vi "Write data file (SubVI).vi"(7 "format (%.;%.7e)":string="%.;%.7e", 8 "error in":errorcluster, 9 "Binary":bool, 10 "2D data":dbl[][](array[numeric]), 11 "file path in":path) -> (0 "error out":errorcluster, 3 "file path out":path)   [LabVIEW 2019]
doc: "Writes measurement data to a file (binary or text based)"
uses:
  <vilib>/Utility/file.llb/Write Delimited Spreadsheet (DBL).vi
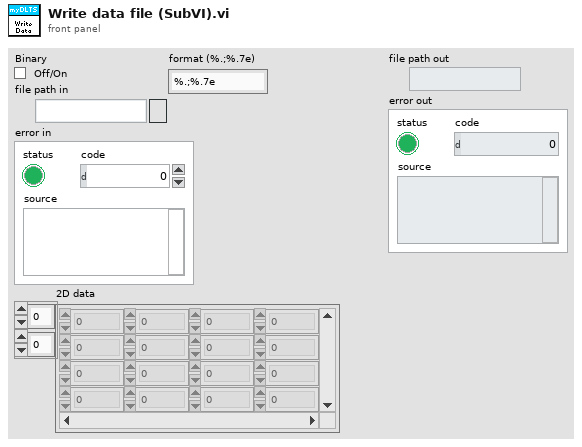
[diagram p1: front panel]
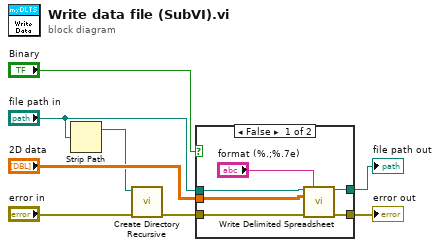
[diagram p0: block diagram]
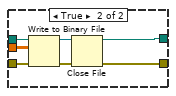
[diagram p2: hidden frame]
diagram:
  n1 = Strip Path(path="file path in") -> (stripped path=w3:path)  [unwired: 1 out]
  n2 = call <vilib>:"Create Directory Recursive.vi"("error in (no error)"="error in", "directory"=w3) -> ("error out"=w1:errorcluster)  [unwired: 3 in, 2 out]
  n3 = case shown="False" "Binary" {
    tunnel: "file path in" -> [w13 w21]
    tunnel: w1 -> [w14 w20]
    tunnel: [w9 w17] -> w6
    tunnel: [w10 w16] -> w7
    tunnel: "2D data" -> [w12 w15]
    frame False {
      n4 = call-poly <vilib>:"Write Delimited Spreadsheet.vi"("file path (dialog if empty)"=w13, "format (%.3f)"="format (%.;%.7e)", "2D data"=w12, "error in (no error)"=w14) -> ("new file path (Not A Path if cancelled)"=w10:path, "error out"=w9:errorcluster)  [unwired: 10 in]
    }
    frame True {
      n5 = Write to Binary File(file (use dialog)=w21, data=w15, error in=w20) -> (refnum out=w19:refnum<file>, error out=w18:errorcluster)  [unwired: 3 in, 1 out]
      n6 = Close File(refnum=w19, error in=w18) -> (path=w16:path, error out=w17:errorcluster)
    }
  }
  "file path out" <- w7
  "error out" <- w6
